vi "Push Border.vi"(9 "Direction":enum16{"N", "E", "S", "W"}(ring), 11 "DVR":refnum<data-value>) -> ()   [LabVIEW 2015, in "Shield Wall.lvclass"]
uses:
  Shield Wall.lvclass
  DVR Cluster.ctl
  SubVIs/Read-Only Globals.vi
  Square/Square.lvclass
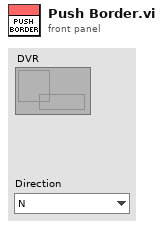
[diagram p1: front panel]
types:
  T1 = typedef "Shield Wall.lvclass/DVR Cluster.ctl" = cluster{"N":i32, "E":i32, "S":i32, "W":i32, "Init":bool, "R":i32}
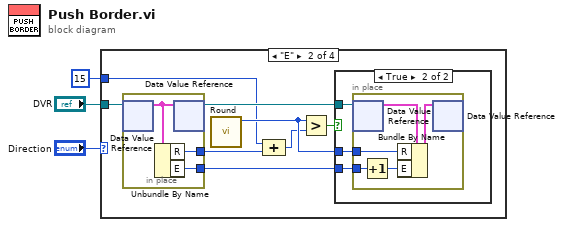
[diagram p0: block diagram]
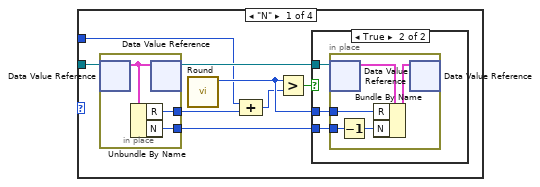
[diagram p2: hidden frame]
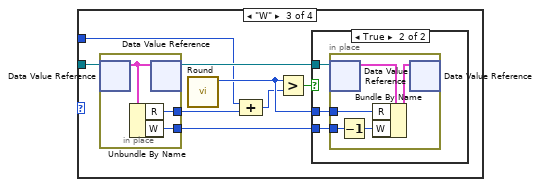
[diagram p5: hidden frame]
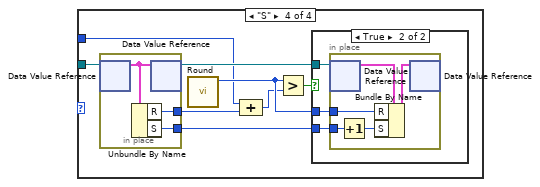
[diagram p7: hidden frame]
diagram:
  n1 = case shown="\"E\"" "Direction" {
    tunnel: "DVR" -> [w11 w30 w49 w68]
    tunnel: 15 ("value") -> [w4 w23 w42 w61]
    frame "N" {
      n2 = in-place {
        in-place-border: [w21] -> w6
        in-place-border: [w20] -> w5
        n3 = in-place-dvr #1(w11) -> (w22:T1)  [unwired: 1 out]
        n4 = Unbundle By Name(w22) -> ("R"=w21:i32, "N"=w20:i32)
        n5 = in-place-dvr #1(w22) -> (w8:refnum<data-value>)  [unwired: 1 out]
      }
      n6 = call "Round.vi"() -> ("Round"=w10:i32)  [unwired: 11 in]
      n7 = Compound Arithmetic op=ADD(w4, w6) -> (w9:i32)
      n8 = Greater?(x=w10, y=w9) -> (0:w7:bool)
      n9 = case shown="True" w7 {
        tunnel: w10 -> [_ w14]
        tunnel: w8 -> [_ w13]
        tunnel: w5 -> [_ w12]
        frame False {
        }
        frame True {
          n10 = in-place {
            in-place-border: w12 -> [w17]
            in-place-border: w14 -> [w15]
            n11 = in-place-dvr #2(w13) -> (w19:T1)  [unwired: 1 out]
            n12 = Decrement(x=w17) -> (x-1=w16:i32)
            n13 = Bundle By Name(cluster=w19, "R"=w15, "N"=w16) -> (w18:T1)
            n14 = in-place-dvr #2(w18) -> ()  [unwired: 2 out]
          }
        }
      }
    }
    frame "E" {
      n15 = in-place {
        in-place-border: [w40] -> w25
        in-place-border: [w39] -> w24
        n16 = in-place-dvr #3(w30) -> (w41:T1)  [unwired: 1 out]
        n17 = Unbundle By Name(w41) -> ("R"=w40:i32, "E"=w39:i32)
        n18 = in-place-dvr #3(w41) -> (w27:refnum<data-value>)  [unwired: 1 out]
      }
      n19 = call "Round.vi"() -> ("Round"=w29:i32)  [unwired: 11 in]
      n20 = Compound Arithmetic op=ADD(w23, w25) -> (w28:i32)
      n21 = Greater?(x=w29, y=w28) -> (0:w26:bool)
      n22 = case shown="True" w26 {
        tunnel: w29 -> [_ w33]
        tunnel: w27 -> [_ w32]
        tunnel: w24 -> [_ w31]
        frame False {
        }
        frame True {
          n23 = in-place {
            in-place-border: w31 -> [w36]
            in-place-border: w33 -> [w34]
            n24 = in-place-dvr #4(w32) -> (w38:T1)  [unwired: 1 out]
            n25 = Increment(x=w36) -> (x+1=w35:i32)
            n26 = Bundle By Name(cluster=w38, "R"=w34, "E"=w35) -> (w37:T1)
            n27 = in-place-dvr #4(w37) -> ()  [unwired: 2 out]
          }
        }
      }
    }
    frame "W" {
      n28 = in-place {
        in-place-border: [w59] -> w44
        in-place-border: [w58] -> w43
        n29 = in-place-dvr #5(w49) -> (w60:T1)  [unwired: 1 out]
        n30 = Unbundle By Name(w60) -> ("R"=w59:i32, "W"=w58:i32)
        n31 = in-place-dvr #5(w60) -> (w46:refnum<data-value>)  [unwired: 1 out]
      }
      n32 = call "Round.vi"() -> ("Round"=w48:i32)  [unwired: 11 in]
      n33 = Compound Arithmetic op=ADD(w42, w44) -> (w47:i32)
      n34 = Greater?(x=w48, y=w47) -> (0:w45:bool)
      n35 = case shown="True" w45 {
        tunnel: w48 -> [_ w52]
        tunnel: w46 -> [_ w51]
        tunnel: w43 -> [_ w50]
        frame False {
        }
        frame True {
          n36 = in-place {
            in-place-border: w50 -> [w55]
            in-place-border: w52 -> [w53]
            n37 = in-place-dvr #6(w51) -> (w57:T1)  [unwired: 1 out]
            n38 = Decrement(x=w55) -> (x-1=w54:i32)
            n39 = Bundle By Name(cluster=w57, "R"=w53, "W"=w54) -> (w56:T1)
            n40 = in-place-dvr #6(w56) -> ()  [unwired: 2 out]
          }
        }
      }
    }
    frame "S" {
      n41 = in-place {
        in-place-border: [w78] -> w63
        in-place-border: [w77] -> w62
        n42 = in-place-dvr #7(w68) -> (w79:T1)  [unwired: 1 out]
        n43 = Unbundle By Name(w79) -> ("R"=w78:i32, "S"=w77:i32)
        n44 = in-place-dvr #7(w79) -> (w65:refnum<data-value>)  [unwired: 1 out]
      }
      n45 = call "Round.vi"() -> ("Round"=w67:i32)  [unwired: 11 in]
      n46 = Compound Arithmetic op=ADD(w61, w63) -> (w66:i32)
      n47 = Greater?(x=w67, y=w66) -> (0:w64:bool)
      n48 = case shown="True" w64 {
        tunnel: w67 -> [_ w71]
        tunnel: w65 -> [_ w70]
        tunnel: w62 -> [_ w69]
        frame False {
        }
        frame True {
          n49 = in-place {
            in-place-border: w69 -> [w74]
            in-place-border: w71 -> [w72]
            n50 = in-place-dvr #8(w70) -> (w76:T1)  [unwired: 1 out]
            n51 = Increment(x=w74) -> (x+1=w73:i32)
            n52 = Bundle By Name(cluster=w76, "R"=w72, "S"=w73) -> (w75:T1)
            n53 = in-place-dvr #8(w75) -> ()  [unwired: 2 out]
          }
        }
      }
    }
  }
